vi "RefMem DMA Main Page.vi"(8 "error in (no error)":errorcluster, 11 "Node Ptr":T1 format="%.0x") -> (0 "error out":errorcluster)   [LabVIEW 2019, in "GE_RM_System Explorer.lvlib"]
uses:
  GE_RM_System Explorer.lvlib
  <vilib>/NI VeriStand/Custom Device API/Custom Device Item Ref.ctl
  <vilib>/NI VeriStand/Custom Device API/Custom Device Execution Mode.ctl
  <vilib>/NI VeriStand/Custom Device API/Path Specification.ctl
  <vilib>/NI VeriStand/Custom Device API/Path Type.ctl
  <vilib>/NI VeriStand/Custom Device API/Custom Device Channel.ctl
  <vilib>/NI VeriStand/Custom Device API/Custom Device Channel Type.ctl
  Shared/Data Channel Type.ctl
  Shared/Global.vi
  <vilib>/NI VeriStand/Custom Device API/Get Item Property (String).vi
  <vilib>/NI VeriStand/Custom Device API/Set Item Property (String).vi
  <vilib>/NI VeriStand/Custom Device API/Get Item Property (I32).vi
  <vilib>/NI VeriStand/Custom Device API/Set Item Property (I32).vi
  <vilib>/NI VeriStand/Custom Device API/Get Item Property (Path).vi
  <vilib>/NI VeriStand/Custom Device API/Set Item Property (U16).vi
  <vilib>/NI VeriStand/Custom Device API/Set Item Property (U32).vi
  <vilib>/NI VeriStand/Custom Device API/Custom Device API.lvlib
  Shared/GE_RM_Shared.lvlib
  <vilib>/NI/NI VeriStand Custom Device Import and Export Tool/ImportExport.lvlib
  <vilib>/NI/NI VeriStand Custom Device Import and Export Tool/File Interface Class/File Interface.lvclass
  <vilib>/NI VeriStand/Custom Device API/Set Item Property (Path).vi
panel:
  out "CSV File Path":path
  out "Version":string
  in  "CPU Assignment":i32
  in  "Import":bool
  in  "Decimation":i32=1 min=1
  in  "VISA Name":string
  in  "Add Data Channel":bool
  in  "Add Data Folder":bool
  in  "Header":cluster{"Section Name":string}={"Section Name"="Reflective Memory Settings"}
  in  "Description":string
  in  "Name":string
  # "(-2 is Automatic)"
  # "Valid values -2, 0, 1.."
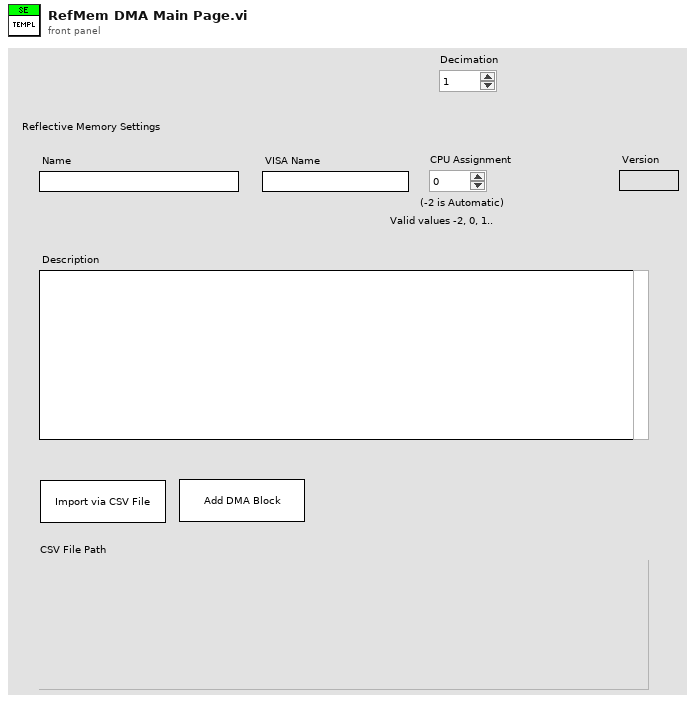
[diagram p1: front panel]
types:
  T1 = typedef "Custom Device API.lvlib/Custom Device Item Ref.ctl" = u64
  T2 = enum8{"Enabled", "Disabled", "Disabled and Grayed Out"}
  T3 = typedef "Custom Device API.lvlib/Custom Device Item Info.ctl" = cluster{"Name":string, "Is Channel":bool, "GUID":string, "Is Waveform":bool}
  T4 = typedef "Custom Device API.lvlib/Path Specification.ctl" = cluster{"Path":path, "Type":T5}
  T5 = typedef "Custom Device API.lvlib/Path Type.ctl" = enum16{"Absolute", "To Base", "To Common Data Dir", "To Application Data Dir"}
  T6 = typedef "Custom Device API.lvlib/Custom Device Execution Mode.ctl" = enum16{"Asynchronous", "Inline HW Interface", "Inline Model Interface", "Inline Timing and Sync", "Asynchronous Timing and Sync"}
  T7 = typedef "GE_RM_System Explorer.lvlib/Data Channel Type.ctl" = enum16{"Read", "Write"}
  T8 = typedef "Custom Device API.lvlib/Custom Device Channel.ctl" = cluster{"Type":T9, "Units":string, "Default Value":dbl, "Faultable":bool, "Scalable":bool}
  T9 = typedef "Custom Device API.lvlib/Custom Device Channel Type.ctl" = enum16{"Input", "Output"}
  T10 = typedef "Custom Device API.lvlib/Custom Device Commands.ctl" = enum16{"Default", "Item renamed", "Shutdown", "Dynamic button pressed"}
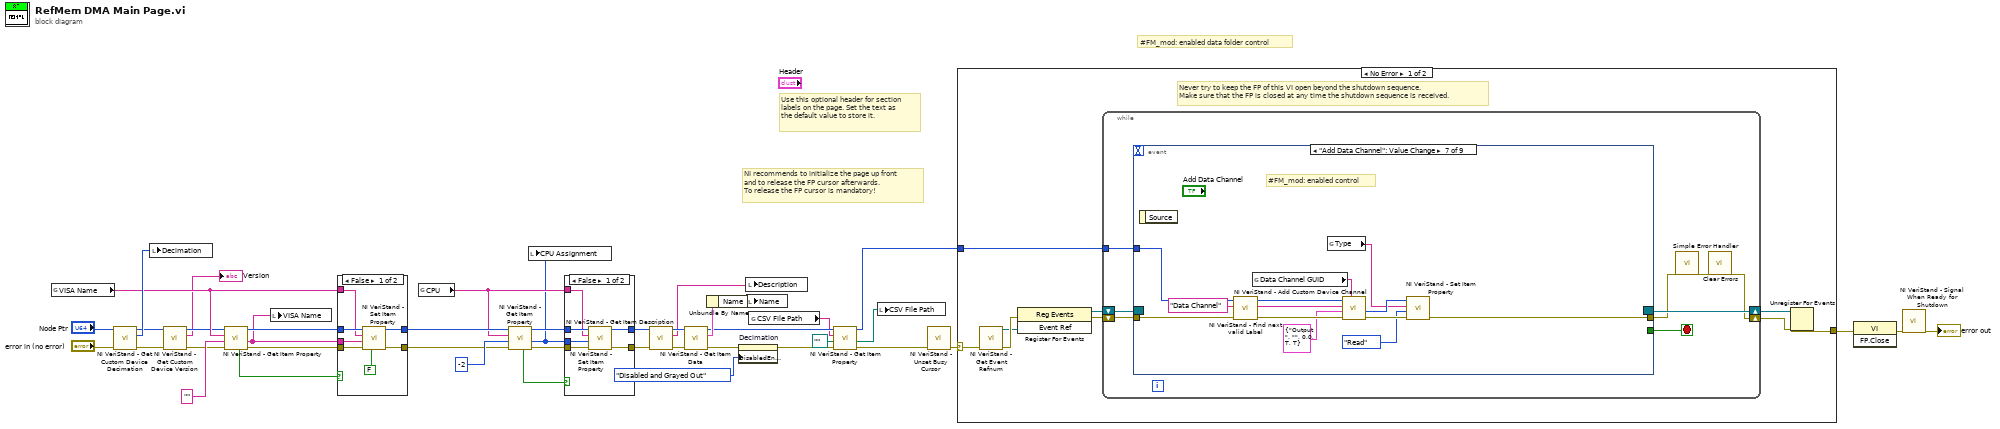
[diagram p0: block diagram]
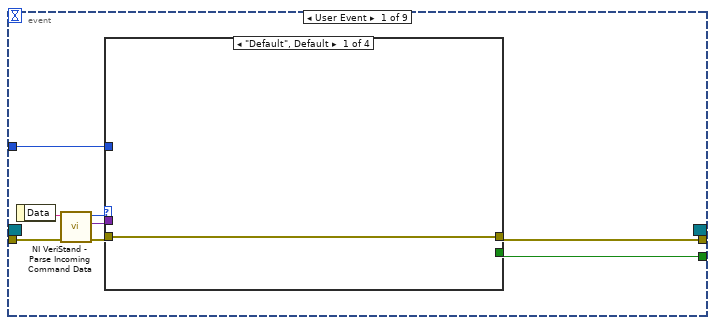
[diagram p4: hidden frame]
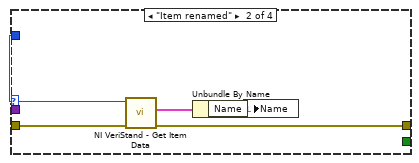
[diagram p5: hidden frame]
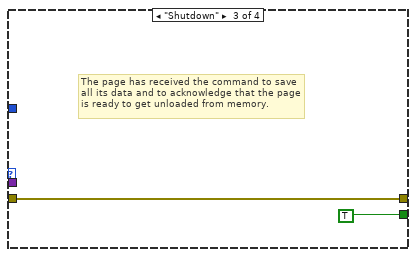
[diagram p6: hidden frame]
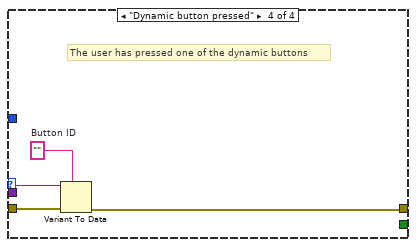
[diagram p7: hidden frame]
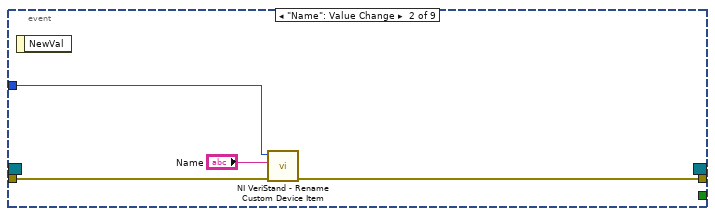
[diagram p8: hidden frame]
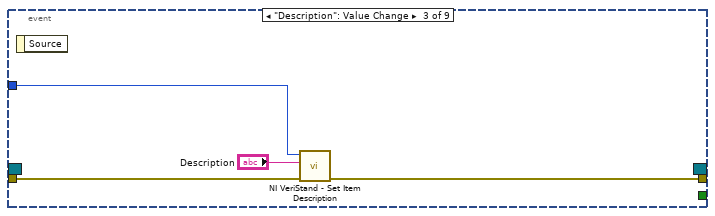
[diagram p9: hidden frame]
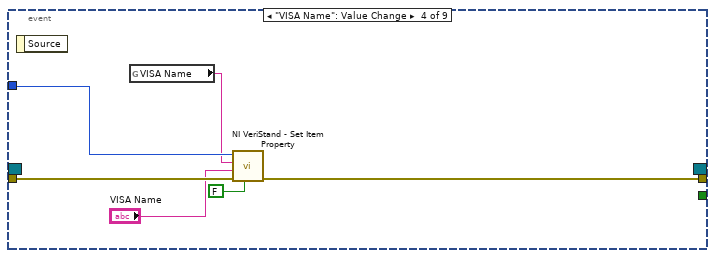
[diagram p10: hidden frame]
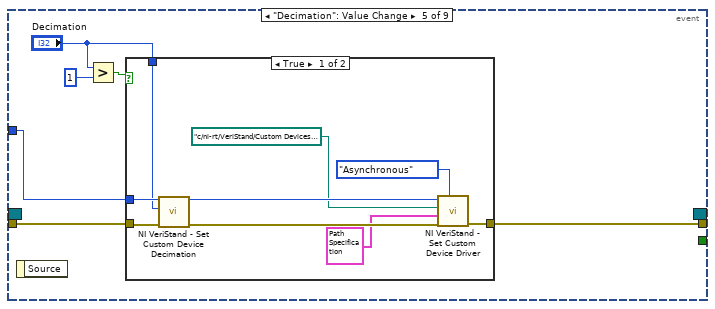
[diagram p11: hidden frame]
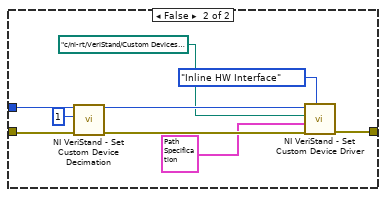
[diagram p12: hidden frame]
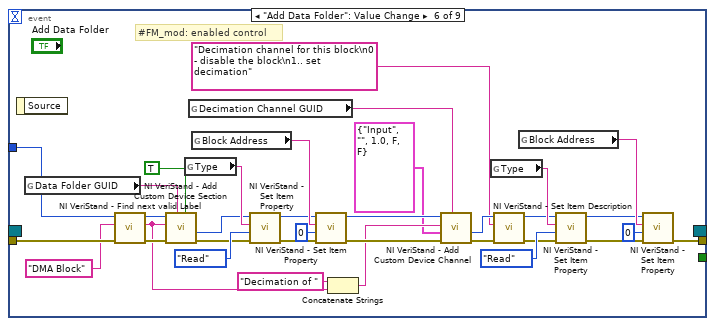
[diagram p13: hidden frame]
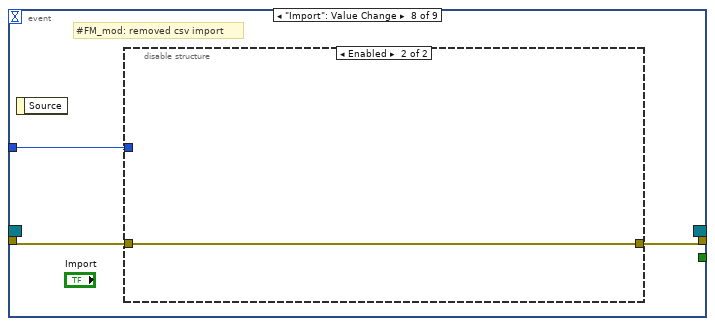
[diagram p14: hidden frame]
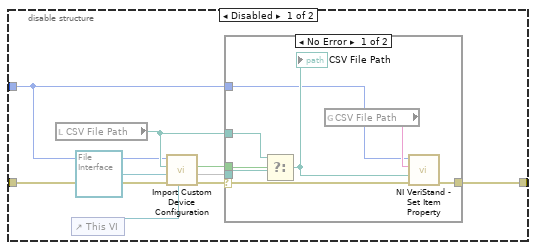
[diagram p15: hidden frame]
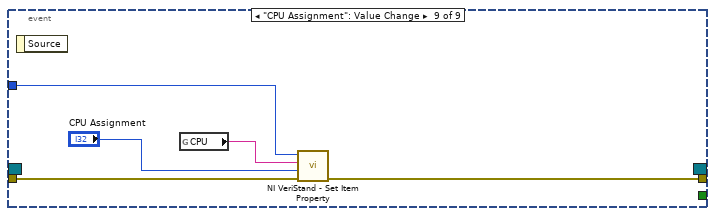
[diagram p17: hidden frame]
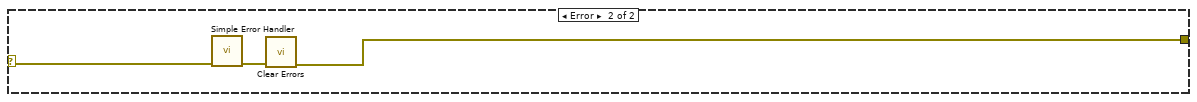
[diagram p18: hidden frame]
diagram:
  # "#FM_mod: enabled data folder control"
  # "Use this optional header for section labels on the page. Set the text as the default value to store it."
  # "NI recommends to initialize the page up front\nand to release the FP cursor afterwards.\nTo release the FP cursor is mandatory!"
  n1 = global read "Global.vi" "VISA Name"() -> (w24:string)
  n2 = call <vilib>:"NI VeriStand - Get Custom Device Decimation.vi"("error in (no error)"="error in (no error)", "Device Ref in"="Node Ptr") -> ("error out"=w11:errorcluster, "Decimation"=w31:i32, "Device Ref out"=w12:T1)  [unwired: 7 in]
  n3 = local write "Decimation"(w31) -> ()
  n4 = call <vilib>:"NI VeriStand - Get Custom Device Version.vi"("error in (no error)"=w11, "Device Ref in"=w12) -> ("error out"=w10:errorcluster, "Value"=→"Version":string, "Device Ref out"=w9:T1)  [unwired: 7 in]
  n5 = call-poly <vilib>:"NI VeriStand - Get Item Property.vi"("error in (no error)"=w10, "Default Value"="" ("Section Name"), "Property Name"=w24, "Item Ref in"=w9) -> ("error out"=w22:errorcluster, "Value"=w23:string, "Item Ref out"=w25:T1, "Found?"=w26:bool)  [unwired: 4 in]
  n6 = local write "VISA Name"(w23) -> ()
  n7 = case shown="False" w26 {
    tunnel: w25 -> [w49 w50]
    tunnel: w24 -> [w48 _]
    tunnel: w23 -> [w47 _]
    tunnel: w22 -> [w46 w51]
    tunnel: [w45 w51] -> w21
    tunnel: [w44 w50] -> w20
    frame False {
      n8 = call-poly <vilib>:"NI VeriStand - Set Item Property.vi"("Binary String (T)"=FALSE, "error in (no error)"=w46, "Value"=w47, "Property Name"=w48, "Item Ref in"=w49) -> ("error out"=w45:errorcluster, "Item Ref out"=w44:T1)  [unwired: 4 in, 1 out]
    }
    frame True {
    }
  }
  n9 = global read "Global.vi" "CPU"() -> (w17:string)
  n10 = call-poly <vilib>:"NI VeriStand - Get Item Property.vi"("error in (no error)"=w21, "Default Value"=-2 ("CPU Assignment"), "Property Name"=w17, "Item Ref in"=w20) -> ("error out"=w18:errorcluster, "Value"=w16:i32, "Item Ref out"=w19:T1, "Found?"=w13:bool)  [unwired: 4 in]
  n11 = local write "CPU Assignment"(w16) -> ()
  n12 = case shown="False" w13 {
    tunnel: w19 -> [w57 w58]
    tunnel: w17 -> [w56 _]
    tunnel: w18 -> [w55 w59]
    tunnel: [w54 w59] -> w14
    tunnel: [w53 w58] -> w15
    tunnel: w16 -> [w52 _]
    frame False {
      n13 = call-poly <vilib>:"NI VeriStand - Set Item Property.vi"("error in (no error)"=w55, "Value"=w52, "Property Name"=w56, "Item Ref in"=w57) -> ("error out"=w54:errorcluster, "Item Ref out"=w53:T1)  [unwired: 5 in, 1 out]
    }
    frame True {
    }
  }
  n14 = call <vilib>:"NI VeriStand - Get Item Description.vi"("error in (no error)"=w14, "Item Ref in"=w15) -> ("error out"=w36:errorcluster, "Description"=w37:string, "Item Ref out"=w38:T1)  [unwired: 7 out]
  n15 = call <vilib>:"NI VeriStand - Get Item Data.vi"("error in (no error)"=w36, "Item Ref in"=w38) -> ("error out"=w28:errorcluster, "Item Info"=w35:T3, "Item Ref out"=w7:T1)  [unwired: 7 out]
  n16 = Unbundle By Name(w35) -> ("Name"=w34:string)
  n17 = property on="Decimation" class="DigNum (strict)"(error in=w28, "DisabledEnum"=T2."Disabled and Grayed Out" ("Disabled")) -> (error out=w6:errorcluster)  [unwired: 1 in, 1 out]
  n18 = local write "Description"(w37) -> ()
  n19 = local write "Name"(w34) -> ()
  n20 = global read "Global.vi" "CSV File Path"() -> (w3:string)
  n21 = call-poly <vilib>:"NI VeriStand - Get Item Property.vi"("error in (no error)"=w6, "Default Value"=path "", "Property Name"=w3, "Item Ref in"=w7) -> ("error out"=w5:errorcluster, "Value"=w1:path, "Item Ref out"=w4:T1)  [unwired: 4 in, 1 out]
  n22 = local write "CSV File Path"(w1) -> ()
  n23 = call <vilib>:"NI VeriStand - Unset Busy Cursor.vi"("error in (no error)"=w5) -> ("error out"=w39:errorcluster)  [unwired: 10 out]
  n24 = case shown="No Error" w39 {
    selector: w39 -> [w61 w211]
    tunnel: [w65 w209] -> w42
    tunnel: w4 -> [w60 _]
    frame No Error {
      # "Never try to keep the FP of this VI open beyond the shutdown sequence.\nMake sure that the FP is closed at any time the shutdown sequence is received."
      n25 = call <vilib>:"NI VeriStand - Get Event Refnum.vi"("error in (no error)"=w61) -> ("error out"=w68:errorcluster, "Event Ref"=w64:refnum<user-event>)  [unwired: 9 out]
      n26 = register-events(error in=w68, w64) -> (reference out=w62:refnum<event-registration>, error out=w63:errorcluster)  [unwired: 1 in]
      n27 = while {
        tunnel: w60 -> [w72]
        shift-right: [w69] -> w66
        shift-left: w63 -> [w75]
        shift-right: [w76] -> w67
        shift-left: w62 -> [w74]
        stop <- w73 stop-if-true
        n28 = event shown="[6] \"Add Data Channel\": Value Change" {
          selector: w74 -> [_ _ _ _ _ _ _ _ _]
          dyn-events: [_ _ _ _ _ _ _ _ _] -> w76
          timeout: _ -> [_ _ _ _ _ _ _ _ _]
          tunnel: w75 -> [w84 w100 w103 w110 w114 w167 w180 w184 w208]
          tunnel: [w80 _ _ _ _ _ _ _ _] -> w73
          tunnel: [w79 w99 w102 w108 w113 w135 w172 w183 w207] -> w71
          tunnel: w72 -> [w78 w98 w104 w109 w112 w166 w179 w182 w205]
          event User Event {
            n29 = event-data() -> ("Data"=w83:string)  [unwired: 1 out]
            n30 = call <vilib>:"NI VeriStand - Parse Incoming Command Data.vi"("error in (no error)"=w84, "Incoming data"=w83) -> ("error out"=w82:errorcluster, "Outgoing data"=w77:variant, "Action"=w81:T10)  [unwired: 7 out]
            n31 = case shown="\"Default\", Default" w81 {
              tunnel: w82 -> [w85 w90 w91 w96]
              tunnel: [_ _ TRUE _] -> w80
              tunnel: [w85 w87 w91 w93] -> w79
              tunnel: w78 -> [_ w89 _ _]
              tunnel: w77 -> [_ _ _ w95]
              frame "Default", Default {
              }
              frame "Item renamed" {
                n32 = call <vilib>:"NI VeriStand - Get Item Data.vi"("error in (no error)"=w90, "Item Ref in"=w89) -> ("error out"=w87:errorcluster, "Item Info"=w88:T3)  [unwired: 8 out]
                n33 = Unbundle By Name(w88) -> ("Name"=w86:string)
                n34 = local write "Name"(w86) -> ()
              }
              frame "Shutdown" {
                # "The page has received the command to save all its data and to acknowledge that the page is ready to get unloaded from memory."
              }
              frame "Dynamic button pressed" {
                w94 = ""  # Button ID
                # "The user has pressed one of the dynamic buttons"
                n35 = Variant To Data(error in=w96, type=w94, Variant=w95) -> (error out=w93:errorcluster)  [unwired: 1 out]
              }
            }
          }
          event "Name": Value Change {
            n36 = event-data() -> ()  [unwired: 2 out]
            n37 = call <vilib>:"NI VeriStand - Rename Custom Device Item.vi"("error in (no error)"=w100, "New Name"="Name", "Item Ref in"=w98) -> ("error out"=w99:errorcluster)  [unwired: 1 in, 7 out]
          }
          event "Description": Value Change {
            n38 = event-data() -> ()  [unwired: 2 out]
            n39 = call <vilib>:"NI VeriStand - Set Item Description.vi"("error in (no error)"=w103, "Description"="Description", "Item Ref in"=w104) -> ("error out"=w102:errorcluster)  [unwired: 8 out]
          }
          event "VISA Name": Value Change {
            n40 = event-data() -> ()  [unwired: 2 out]
            n41 = global read "Global.vi" "VISA Name"() -> (w106:string)
            n42 = call-poly <vilib>:"NI VeriStand - Set Item Property.vi"("Binary String (T)"=FALSE, "error in (no error)"=w110, "Value"="VISA Name", "Property Name"=w106, "Item Ref in"=w109) -> ("error out"=w108:errorcluster)  [unwired: 4 in, 2 out]
          }
          event "Decimation": Value Change {
            n43 = event-data() -> ()  [unwired: 2 out]
            n44 = Greater?(x="Decimation", y=u32 1) -> (0:w115:bool)
            n45 = case shown="True" w115 {
              tunnel: w114 -> [w123 w132]
              tunnel: [w125 w134] -> w113
              tunnel: w112 -> [w122 w131]
              tunnel: "Decimation" -> [w121 _]
              frame True {
                n46 = call <vilib>:"NI VeriStand - Set Custom Device Decimation.vi"("error in (no error)"=w123, "Decimation"=w121, "Device Ref in"=w122) -> ("error out"=w120:errorcluster, "Device Ref out"=w119:T1)  [unwired: 7 in]
                n47 = call <vilib>:"NI VeriStand - Set Custom Device Driver.vi"("Execution mode"=Custom_Device_Execution_Mode."Asynchronous", "error in (no error)"=w120, "Driver VI Path (Host)"=T4 {"Path"=path "Custom Devices/RefMem PtByPt/RefMem PtByPt Engine.llb/RefMem PtByPt RT Driver VI (Async).vi", "Type"=enum."To Common Data Dir"}, "Driver VI Path (RT)"=path "c:/ni-rt/VeriStand/Custom Devices/RefMem PtByPt/RefMem PtByPt Engine.llb/RefMem PtByPt RT Driver VI (Async).vi", "Device Ref in"=w119) -> ("error out"=w125:errorcluster)  [unwired: 5 in, 1 out]
              }
              frame False {
                n48 = call <vilib>:"NI VeriStand - Set Custom Device Decimation.vi"("error in (no error)"=w132, "Decimation"=1, "Device Ref in"=w131) -> ("error out"=w130:errorcluster, "Device Ref out"=w129:T1)  [unwired: 7 in]
                n49 = call <vilib>:"NI VeriStand - Set Custom Device Driver.vi"("Execution mode"=Custom_Device_Execution_Mode."Inline HW Interface", "error in (no error)"=w130, "Driver VI Path (Host)"=T4 {"Path"=path "Custom Devices/RefMem PtByPt/RefMem PtByPt Engine.llb/RefMem PtByPt RT Driver VI (Inline).vi", "Type"=enum."To Common Data Dir"}, "Driver VI Path (RT)"=path "c:/ni-rt/VeriStand/Custom Devices/RefMem PtByPt/RefMem PtByPt Engine.llb/RefMem PtByPt RT Driver VI (Inline).vi", "Device Ref in"=w129) -> ("error out"=w134:errorcluster)  [unwired: 5 in, 1 out]
              }
            }
          }
          event "Add Data Folder": Value Change {
            # "#FM_mod: enabled control"
            n50 = event-data() -> ()  [unwired: 2 out]
            n51 = global read "Global.vi" "Data Folder GUID"() -> (w168:string)
            n52 = call <vilib>:"NI VeriStand - Find next valid Label.vi"("error in (no error)"=w167, "Label"="DMA Block" ("Section Name"), "Item Ref in"=w166) -> ("error out"=w163:errorcluster, "Label out"=w151:string, "Item Ref out"=w165:T1)  [unwired: 4 in, 2 out]
            n53 = call <vilib>:"NI VeriStand - Add Custom Device Section.vi"("Highlight? (F)"=TRUE, "GUID (Default Section)"=w168, "error in (no error)"=w163, "Section Name"=w151, "Parent Ref in"=w165) -> ("error out"=w159:errorcluster, "Section Ptr"=w154:T1)  [unwired: 3 in, 2 out]
            n54 = global read "Global.vi" "Type"() -> (w161:string)
            n55 = global read "Global.vi" "Decimation Channel GUID"() -> (w149:string)
            n56 = global read "Global.vi" "Block Address"() -> (w162:string)
            n57 = call-poly <vilib>:"NI VeriStand - Set Item Property.vi"("error in (no error)"=w159, "Value"=Data_Channel_Type."Read" ("Type"), "Property Name"=w161, "Item Ref in"=w154) -> ("error out"=w157:errorcluster, "Item Ref out"=w156:T1)  [unwired: 5 in, 1 out]
            n58 = call-poly <vilib>:"NI VeriStand - Set Item Property.vi"("error in (no error)"=w157, "Value"=u32 0 ("Default Value"), "Property Name"=w162, "Item Ref in"=w156) -> ("error out"=w155:errorcluster, "Item Ref out"=w153:T1)  [unwired: 5 in, 1 out]
            n59 = Concatenate Strings("Decimation of " ("string"), w151) -> (w150:string)
            n60 = call <vilib>:"NI VeriStand - Add Custom Device Channel.vi"("GUID (Default Channel)"=w149, "error in (no error)"=w155, "Channel"=T8 {"Type"=enum."Input", "Units"="", "Default Value"=1.0, "Faultable"=FALSE, "Scalable"=FALSE}, "Channel Name"=w150, "Parent Ref in"=w153) -> ("error out"=w147:errorcluster, "Channel Ref"=w146:T1)  [unwired: 3 in, 2 out]
            n61 = global read "Global.vi" "Type"() -> (w142:string)
            n62 = call <vilib>:"NI VeriStand - Set Item Description.vi"("error in (no error)"=w147, "Description"="Decimation channel for this block\n0 - disable the block\n1.. set decimation" ("Section Name"), "Item Ref in"=w146) -> ("error out"=w141:errorcluster, "Item Ref out"=w140:T1)  [unwired: 6 in, 1 out]
            n63 = global read "Global.vi" "Block Address"() -> (w138:string)
            n64 = call-poly <vilib>:"NI VeriStand - Set Item Property.vi"("error in (no error)"=w141, "Value"=Data_Channel_Type."Read" ("Type"), "Property Name"=w142, "Item Ref in"=w140) -> ("error out"=w136:errorcluster, "Item Ref out"=w137:T1)  [unwired: 5 in, 1 out]
            n65 = call-poly <vilib>:"NI VeriStand - Set Item Property.vi"("error in (no error)"=w136, "Value"=u32 0 ("Default Value"), "Property Name"=w138, "Item Ref in"=w137) -> ("error out"=w135:errorcluster)  [unwired: 5 in, 2 out]
          }
          event "Add Data Channel": Value Change {
            # "#FM_mod: enabled control"
            n66 = event-data() -> ()  [unwired: 2 out]
            n67 = call <vilib>:"NI VeriStand - Find next valid Label.vi"("error in (no error)"=w180, "Label"="Data Channel", "Item Ref in"=w179) -> ("error out"=w176:errorcluster, "Label out"=w178:string, "Item Ref out"=w177:T1)  [unwired: 4 in, 2 out]
            n68 = global read "Global.vi" "Data Channel GUID"() -> (w181:string)
            n69 = global read "Global.vi" "Type"() -> (w170:string)
            n70 = call <vilib>:"NI VeriStand - Add Custom Device Channel.vi"("GUID (Default Channel)"=w181, "error in (no error)"=w176, "Channel"=T8 {"Type"=enum."Output", "Units"="", "Default Value"=0.0, "Faultable"=TRUE, "Scalable"=TRUE}, "Channel Name"=w178, "Parent Ref in"=w177) -> ("error out"=w173:errorcluster, "Channel Ref"=w171:T1)  [unwired: 3 in, 2 out]
            n71 = call-poly <vilib>:"NI VeriStand - Set Item Property.vi"("error in (no error)"=w173, "Value"=Data_Channel_Type."Read" ("Type"), "Property Name"=w170, "Item Ref in"=w171) -> ("error out"=w172:errorcluster)  [unwired: 5 in, 2 out]
          }
          event "Import": Value Change {
            # "#FM_mod: removed csv import"
            n72 = event-data() -> ()  [unwired: 2 out]
            n73 = disable-structure shown="Enabled" {
              disable-tunnel: w184 -> [w193 w203]
              disable-tunnel: [w189 w203] -> w183
              disable-tunnel: w182 -> [w185 _]
              frame Disabled {
                n74 = local read "CSV File Path"() -> (w188:path)
                n75 = control-ref of="This VI"() -> (w191:refnum<vi>)
                n76 = call <vilib>:"Import Custom Device Configuration.vi"(6:w191, "error in (no error)"=w193, "File Interface (.dat)"=refnum<class "File Interface.lvclass"> refnum, "Path"=w188, "NodeID"=w185) -> ("error out"=w190:errorcluster, 1:w187, "cancelled"=w186:bool)  [unwired: 3 in, 1 out]
                n77 = case shown="No Error" w190 {
                  selector: w190 -> [w197 w202]
                  tunnel: [w196 w202] -> w189
                  tunnel: w188 -> [w200 _]
                  tunnel: w187 -> [w199 _]
                  tunnel: w186 -> [w201 _]
                  tunnel: w185 -> [w194 _]
                  frame No Error {
                    n78 = Select(t=w200, s=w201, f=w199) -> (s? t:f=w195:path)
                    "CSV File Path" <- w195
                    n79 = global read "Global.vi" "CSV File Path"() -> (w198:string)
                    n80 = call-poly <vilib>:"NI VeriStand - Set Item Property.vi"("error in (no error)"=w197, "Value"=w195, "Property Name"=w198, "Item Ref in"=w194) -> ("error out"=w196:errorcluster)  [unwired: 5 in, 2 out]
                  }
                  frame Error {
                  }
                }
              }
              frame Enabled {
              }
            }
          }
          event "CPU Assignment": Value Change {
            n81 = event-data() -> ()  [unwired: 2 out]
            n82 = global read "Global.vi" "CPU"() -> (w206:string)
            n83 = call-poly <vilib>:"NI VeriStand - Set Item Property.vi"("error in (no error)"=w208, "Value"="CPU Assignment", "Property Name"=w206, "Item Ref in"=w205) -> ("error out"=w207:errorcluster)  [unwired: 5 in, 2 out]
          }
        }
        n84 = call <vilib>:"Simple Error Handler.vi"("error in (no error)"=w71) -> ("error out"=w70:errorcluster)  [unwired: 1 in, 7 out]
        n85 = call <vilib>:"Clear Errors.vi"("error in (no error)"=w70) -> ("error out"=w69:errorcluster)  [unwired: 1 in, 5 out]
      }
      n86 = Unregister For Events(event registration refnum=w67, error in=w66) -> (error out=w65:errorcluster)
    }
    frame Error {
      n87 = call <vilib>:"Simple Error Handler.vi"("error in (no error)"=w211) -> ("error out"=w210:errorcluster)  [unwired: 1 in, 7 out]
      n88 = call <vilib>:"Clear Errors.vi"("error in (no error)"=w210) -> ("error out"=w209:errorcluster)  [unwired: 1 in, 5 out]
    }
  }
  n89 = invoke class="VI" method="FP.Close"(error in=w42) -> (error out=w41:errorcluster)  [unwired: 2 in, 2 out]
  n90 = call <vilib>:"NI VeriStand - Signal When Ready for Shutdown.vi"("error in (no error)"=w41) -> ("error out"=→"error out":errorcluster)  [unwired: 10 out]
